vi "Global_grid settings.vi"() -> ()   [LabVIEW 2012]
panel:
  in  "Grid Settings":T1
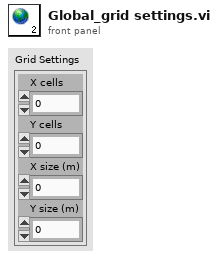
[diagram p1: front panel]
types:
  T1 = cluster{"X cells":i32, "Y cells":i32, "X size (m)":dbl, "Y size (m)":dbl}
diagram:
